vi "Function.vi"(8 "error in (no error)":errorcluster, 10 "Value":sgl, 11 "Two Terminal in":refnum<class "Decrement_SGL.lvclass">) -> (0 "error out":errorcluster, 2 "Result":sgl, 3 "Two Terminal out":refnum<class "Decrement_SGL.lvclass">)   [LabVIEW 2021, in "Decrement_SGL.lvclass"]
uses:
  Decrement_SGL.lvclass
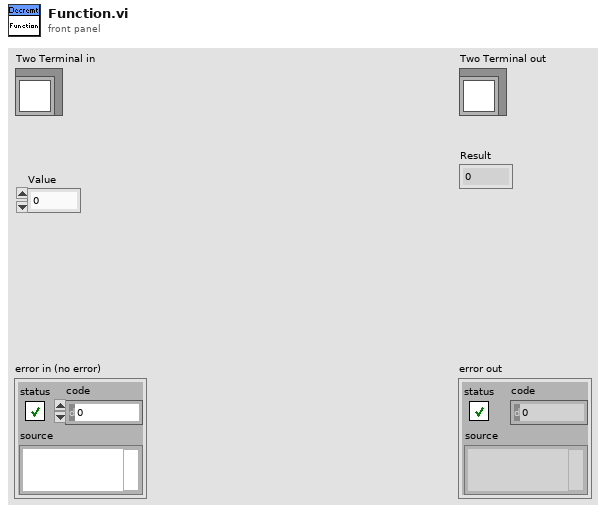
[diagram p1: front panel]
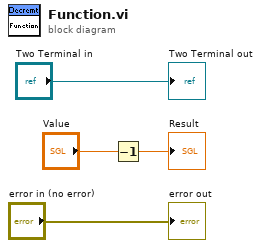
[diagram p0: block diagram]
diagram:
  n1 = Decrement(x="Value") -> (x-1=→"Result":sgl)
  "error out" <- "error in (no error)"
  "Two Terminal out" <- "Two Terminal in"
